vi "Clear All Buffers.vi"(8 "error in (no error)":errorcluster, 11 "Collection.lvclass In":refnum<class "Collection.lvclass">) -> (0 "error Out":errorcluster, 3 "Collection.lvclass Out":refnum<class "Collection.lvclass">)   [LabVIEW 2012, in "Collection.lvclass"]
uses:
  Collection.lvclass
  Collection.lvclass/Collection.ctl
  Readable/Readable.lvclass
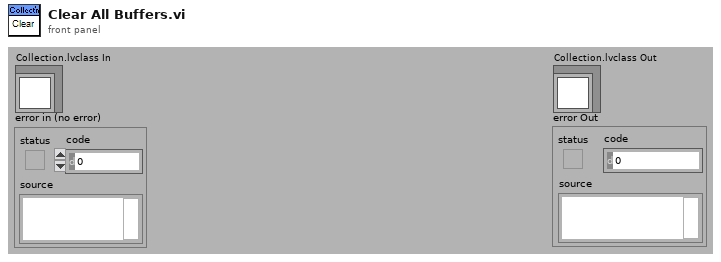
[diagram p1: front panel]
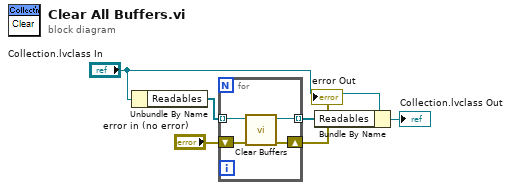
[diagram p0: block diagram]
diagram:
  n1 = Unbundle By Name("Collection.lvclass In") -> ("Readables"=w6:refnum<class "Readable.lvclass">[])
  n2 = for {
    tunnel: w6 -> [w10] mode=indexing
    shift-right: [w8] -> w1
    shift-left: "error in (no error)" -> [w9]
    tunnel: [w7] -> w3 mode=indexing
    n3 = call "Clear Buffers.vi"("error in (no error)"=w9, "Readable in"=w10) -> ("error out"=w8:errorcluster, "Readable out"=w7:refnum<class "Readable.lvclass">)  [unwired: 8 in]
  }
  "error Out" <- w1
  n4 = Bundle By Name(cluster="Collection.lvclass In", "Readables"=w3) -> (→"Collection.lvclass Out":refnum<class "Collection.lvclass">)
